vi "feu.vi"() -> ()   [LabVIEW 2025]
panel:
  in  "sw1":bool
  out "vert":bool
  out "orange":bool
  out "rouge":bool
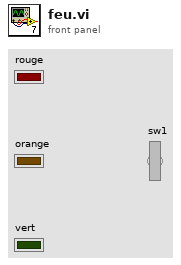
[diagram p1: front panel]
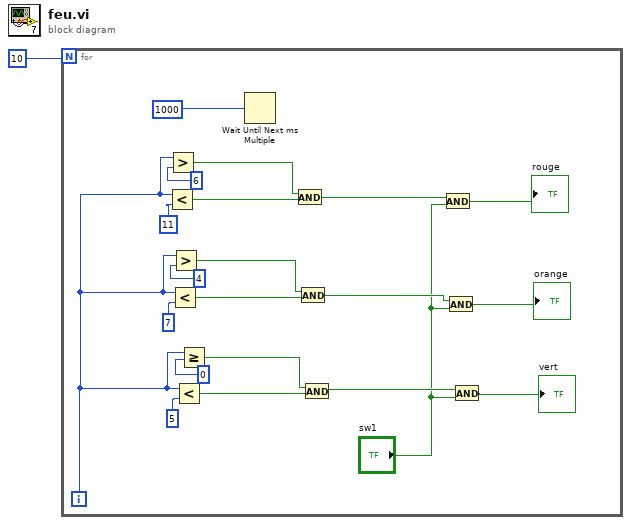
[diagram p0: block diagram]
diagram:
  n1 = for {
    N: 10 -> [_]
    i -> [w10]
    n2 = Less?(x=w10, y=11) -> (x < y?=w15:bool)
    n3 = Greater?(x=w10, y=6) -> (0:w13:bool)
    n4 = Less?(x=w10, y=7) -> (x < y?=w19:bool)
    n5 = Greater?(x=w10, y=4) -> (0:w17:bool)
    n6 = Less?(x=w10, y=5) -> (x < y?=w21:bool)
    n7 = Greater Or Equal?(x=w10, y=0) -> (x >= y?=w11:bool)
    n8 = Wait Until Next ms Multiple(millisecond multiple=1000) -> ()  [unwired: 1 out]
    n9 = And(x=w13, y=w15) -> (x .and. y?=w5:bool)
    n10 = And(x=w17, y=w19) -> (x .and. y?=w4:bool)
    n11 = And(x=w11, y=w21) -> (x .and. y?=w3:bool)
    n12 = And(x=w5, y="sw1") -> (x .and. y?=→"rouge":bool)
    n13 = And(x=w4, y="sw1") -> (x .and. y?=→"orange":bool)
    n14 = And(x=w3, y="sw1") -> (x .and. y?=→"vert":bool)
  }
